vi "符合分析1.4.vi"(5 "大于信号周期":dbl, 6 "length":dbl=60.0 format="%#_13g", 7 "小于信号周期":dbl=120000.0, 8 "min bin":i32=30, 9 "通道B":i32=7, 10 "通道A":i32=6, 11 "file path (dialog if empty)":path=path "D:/tdc/2017/TDC_.fee01._20240514_102433.noAmp_-30mV_multiple_csv.csv") -> (0 "abnormal":bool=TRUE, 1 "Fitting RMS":dbl=2818.43112473961, 2 "Fitting center":dbl=-2250.0, 3 "mean":dbl=-3850.769384392631 format="%0.2f")   [LabVIEW 2017]
uses:
  <vilib>/Utility/file.llb/Read Delimited Spreadsheet (DBL).vi
  <vilib>/Analysis/NI_AALBase.lvlib
panel:
  out "Numeric 2":dbl=5.712308982040112e+16 format="%#_20f"
  out "Numeric":dbl=5.7122985833787944e+16 format="%#_20f"
  out "数值":i32=308738
  out "大小":i32=129310
  out "Histogram 2":dynamicdata(graph)=[{"t0"=timestamp(25 s since 1904-01-01), "dt"=50.0, "Y"=array[20000 elements], "attributes"=variant("NI_ChannelName"=variant(string " (直方图)"), "NI_ExpIsRelativeTime"=variant(bool TRUE), "NI_ExpStartTimeStamp"=variant(timestamp timestamp(3799126030.6251626 s since 1904-01-01)), "NI_ExpTimeStamp"=variant(timestamp timestamp(3799126030.6251626 s since 1904-01-01)), "NI_ExpXDimension"=variant(string "BIN"), "NI_OriginalChannelName"=variant(string ""))}] caption="直方图"
  out "数组":dbl[](array[numeric])
  out "Waveform Graph 5":dbl[](graph)
  in  "禁用的索引 (列)":i32=1
  in  "window":dbl=10000.0 format="%#_13g"
  in  "intervals":i32=200
  in  "min":dbl=-50000.0 format="%#_13g"
  in  "max":dbl=50000.0 format="%#_13g"
  out "XY Graph":cluster{"X":dbl, "Y":dbl}[](graph)
  out "list":dbl[][](array[numeric])
  out "counter":dbl[](array[numeric])=[139102.0, 129310.0, 0.0, 0.0, 0.0, 0.0, 20298.0, 20029.0, 0.0, 0.0, 0.0, 0.0, 0.0, 0.0, 0.0, 0.0, 0.0, 0.0, 0.0, 0.0, 0.0, 0.0, 0.0, 0.0, 0.0, 0.0, 0.0, 0.0, 0.0, 0.0, 0.0, 0.0, 0.0, 0.0, 0.0, 0.0, 0.0, 0.0, 0.0, 0.0, 0.0, 0.0, 0.0, 0.0, 0.0, 0.0, 0.0, 0.0, 0.0, 0.0, 0.0, 0.0, 0.0, 0.0, 0.0, 0.0, 0.0, 0.0, 0.0, 0.0, 0.0, 0.0, 0.0, 0.0]
  out "size(s) 2":i32[](array[numeric])=[308739, 128]
  out "Waveform Graph 4":dbl[](graph)
  out "B_start":i32
  out "A_start":i32
  out "start":i32
  out "mean 2":dbl=-3580.325380501851 format="%0.2f"
  out "standard deviation 2":dbl=2102.674360008159 format="%0.2f"
  out "Sum of 3 Gaussians 2":T1(graph)=[{"X Values"=[-13750.0, -13250.0, -12750.0, -12250.0, -11750.0, -11250.0, -10750.0, -10250.0, -9750.0, -9250.0, -8750.0, -8250.0, -7750.0, -7250.0, -6750.0, -6250.0, -5750.0, -5250.0, -4750.0, -4250.0, -3750.0, -3250.0, -2750.0, -2250.0, -1750.0, -1250.0, -750.0, -250.0, 250.0, 750.0, 1250.0, 1750.0, 2250.0, 2750.0, 3250.0, 3750.0, 4250.0, 4750.0, 5250.0, 5750.0, 6250.0, 6750.0, 7250.0, 7750.0, 8250.0, 8750.0, 9250.0, 9750.0, 10250.0, 10750.0, 11250.0, 11750.0, 12250.0, 12750.0, 13250.0, 13750.0, 14250.0, 14750.0, 15250.0, 15750.0], "Histogram: h(x)"=[0.00020516896563452846, 0.0005879803951743795, 0.00162597544504643, 0.004338754526689241, 0.011171619539264068, 0.027756656713886607, 0.06654541404560899, 0.1539462339582165, 0.34365286320062033, 0.7402370601310521, 1.538585524549578, 3.0858330069334388, 5.972046190316014, 11.152541711235395, 20.096689123234196, 34.94420244889411, 58.63078530864886, 94.92404789337367, 148.2950819797982, 223.55130384724364, 325.18284479713714, 456.43401817417424, 618.1990653887884, 807.9391318829133, 1018.8937603390267, 1239.87847954737, 1455.892475846031, 1649.6030130849056, 1803.555623444127, 1902.740668671416, 1937.0, 1902.740668671416, 1803.555623444127, 1649.6030130849056, 1455.892475846031, 1239.87847954737, 1018.8937603390267, 807.9391318829133, 618.1990653887884, 456.43401817417424, 325.18284479713714, 223.55130384724364, 148.2950819797982, 94.92404789337367, 58.63078530864886, 34.94420244889411, 20.096689123234196, 11.152541711235395, 5.972046190316014, 3.0858330069334388, 1.538585524549578, 0.7402370601310521, 0.34365286320062033, 0.1539462339582165, 0.06654541404560899, 0.027756656713886607, 0.011171619539264068, 0.004338754526689241, 0.00162597544504643, 0.0005879803951743795]}, {"X Values"=[-49750.0, -49250.0, -48750.0, -48250.0, -47750.0, -47250.0, -46750.0, -46250.0, -45750.0, -45250.0, -44750.0, -44250.0, -43750.0, -43250.0, -42750.0, -42250.0, -41750.0, -41250.0, -40750.0, -40250.0, -39750.0, -39250.0, -38750.0, -38250.0, -37750.0, -37250.0, -36750.0, -36250.0, -35750.0, -35250.0, -34750.0, -34250.0, -33750.0, -33250.0, -32750.0, -32250.0, -31750.0, -31250.0, -30750.0, -30250.0, -29750.0, -29250.0, -28750.0, -28250.0, -27750.0, -27250.0, -26750.0, -26250.0, -25750.0, -25250.0, -24750.0, -24250.0, -23750.0, -23250.0, -22750.0, -22250.0, -21750.0, -21250.0, -20750.0, -20250.0, -19750.0, -19250.0, -18750.0, -18250.0, -17750.0, -17250.0, -16750.0, -16250.0, -15750.0, -15250.0, -14750.0, -14250.0, -13750.0, -13250.0, -12750.0, -12250.0, -11750.0, -11250.0, -10750.0, -10250.0, -9750.0, -9250.0, -8750.0, -8250.0, -7750.0, -7250.0, -6750.0, -6250.0, -5750.0, -5250.0, -4750.0, -4250.0, -3750.0, -3250.0, -2750.0, -2250.0, -1750.0, -1250.0, -750.0, -250.0, 250.0, 750.0, 1250.0, 1750.0, 2250.0, 2750.0, 3250.0, 3750.0, 4250.0, 4750.0, 5250.0, 5750.0, 6250.0, 6750.0, 7250.0, 7750.0, 8250.0, 8750.0, 9250.0, 9750.0, 10250.0, 10750.0, 11250.0, 11750.0, 12250.0, 12750.0, 13250.0, 13750.0, 14250.0, 14750.0, 15250.0, 15750.0, 16250.0, 16750.0, 17250.0, 17750.0, 18250.0, 18750.0, 19250.0, 19750.0, 20250.0, 20750.0, 21250.0, 21750.0, 22250.0, 22750.0, 23250.0, 23750.0, 24250.0, 24750.0, 25250.0, 25750.0, 26250.0, 26750.0, 27250.0, 27750.0, 28250.0, 28750.0, 29250.0, 29750.0, 30250.0, 30750.0, 31250.0, 31750.0, 32250.0, 32750.0, 33250.0, 33750.0, 34250.0, 34750.0, 35250.0, 35750.0, 36250.0, 36750.0, 37250.0, 37750.0, 38250.0, 38750.0, 39250.0, 39750.0, 40250.0, 40750.0, 41250.0, 41750.0, 42250.0, 42750.0, 43250.0, 43750.0, 44250.0, 44750.0, 45250.0, 45750.0, 46250.0, 46750.0, 47250.0, 47750.0, 48250.0, 48750.0, 49250.0, 49750.0], "Histogram: h(x)"=[0.0, 0.0, 0.0, 0.0, 0.0, 0.0, 0.0, 0.0, 0.0, 0.0, 0.0, 0.0, 0.0, 0.0, 0.0, 0.0, 0.0, 0.0, 0.0, 0.0, 0.0, 0.0, 0.0, 0.0, 0.0, 0.0, 0.0, 0.0, 0.0, 0.0, 0.0, 0.0, 0.0, 0.0, 0.0, 0.0, 0.0, 0.0, 0.0, 0.0, 0.0, 0.0, 0.0, 0.0, 0.0, 0.0, 0.0, 0.0, 0.0, 0.0, 0.0, 0.0, 0.0, 0.0, 0.0, 0.0, 0.0, 0.0, 0.0, 0.0, 0.0, 0.0, 0.0, 0.0, 0.0, 0.0, 0.0, 0.0, 0.0, 0.0, 0.0, 0.0, 0.0, 0.0, 0.0, 0.0, 0.0, 0.0, 0.0, 0.0, 0.0, 0.0, 0.0, 0.0, 0.0, 0.0, 0.0, 134.0, 159.0, 231.0, 266.0, 307.0, 362.0, 464.0, 641.0, 831.0, 939.0, 1186.0, 1365.0, 1561.0, 1704.0, 1905.0, 1937.0, 1897.0, 1825.0, 1421.0, 313.0, 0.0, 0.0, 0.0, 0.0, 0.0, 0.0, 0.0, 0.0, 0.0, 0.0, 0.0, 0.0, 0.0, 0.0, 0.0, 0.0, 0.0, 0.0, 0.0, 0.0, 0.0, 0.0, 0.0, 0.0, 0.0, 0.0, 0.0, 0.0, 0.0, 0.0, 0.0, 0.0, 0.0, 0.0, 0.0, 0.0, 0.0, 0.0, 0.0, 0.0, 0.0, 0.0, 0.0, 0.0, 0.0, 0.0, 0.0, 0.0, 0.0, 0.0, 0.0, 0.0, 0.0, 0.0, 0.0, 0.0, 0.0, 0.0, 0.0, 0.0, 0.0, 0.0, 0.0, 0.0, 0.0, 0.0, 0.0, 0.0, 0.0, 0.0, 0.0, 0.0, 0.0, 0.0, 0.0, 0.0, 0.0, 0.0, 0.0, 0.0, 0.0, 0.0, 0.0, 0.0, 0.0, 0.0, 0.0, 0.0, 0.0, 0.0, 0.0, 0.0, 0.0]}]
  out "Fitting center 2":dbl=1250.0
  out "Fitting RMS 2":dbl=2646.6453634414506
  in  "min bin 2":i32=30
  in  "length 2":dbl=60.0 format="%#_13g"
  out "Waveform Graph 3":dbl[](graph)
  out "Waveform Graph 2":dbl[](graph)
  out "Sum of 3 Gaussians":T1(graph)=[{"X Values"=[-17250.0, -16750.0, -16250.0, -15750.0, -15250.0, -14750.0, -14250.0, -13750.0, -13250.0, -12750.0, -12250.0, -11750.0, -11250.0, -10750.0, -10250.0, -9750.0, -9250.0, -8750.0, -8250.0, -7750.0, -7250.0, -6750.0, -6250.0, -5750.0, -5250.0, -4750.0, -4250.0, -3750.0, -3250.0, -2750.0, -2250.0, -1750.0, -1250.0, -750.0, -250.0, 250.0, 750.0, 1250.0, 1750.0, 2250.0, 2750.0, 3250.0, 3750.0, 4250.0, 4750.0, 5250.0, 5750.0, 6250.0, 6750.0, 7250.0, 7750.0, 8250.0, 8750.0, 9250.0, 9750.0, 10250.0, 10750.0, 11250.0, 11750.0, 12250.0], "Histogram: h(x)"=[0.0013656626400436554, 0.003455839817507884, 0.008474140067424075, 0.020135829745501498, 0.0463634004710291, 0.10344580667038393, 0.2236569294966776, 0.46857993149481575, 0.9512986254154174, 1.8714658745731036, 3.5676218402583713, 6.590336255723455, 11.796907998790784, 20.46259315061705, 34.39418356941237, 56.01975417683496, 88.41567178978539, 135.22256256877975, 200.4014830434576, 287.7958710191195, 400.4977172476056, 540.0666872618658, 705.7105220811543, 893.5886714395316, 1096.4291526227148, 1303.6330216489944, 1501.9725298165247, 1676.8742089667392, 1814.140166258101, 1901.8359447148478, 1932.0, 1901.8359447148478, 1814.140166258101, 1676.8742089667392, 1501.9725298165247, 1303.6330216489944, 1096.4291526227148, 893.5886714395316, 705.7105220811543, 540.0666872618658, 400.4977172476056, 287.7958710191195, 200.4014830434576, 135.22256256877975, 88.41567178978539, 56.01975417683496, 34.39418356941237, 20.46259315061705, 11.796907998790784, 6.590336255723455, 3.5676218402583713, 1.8714658745731036, 0.9512986254154174, 0.46857993149481575, 0.2236569294966776, 0.10344580667038393, 0.0463634004710291, 0.020135829745501498, 0.008474140067424075, 0.003455839817507884]}, {"X Values"=[-49750.0, -49250.0, -48750.0, -48250.0, -47750.0, -47250.0, -46750.0, -46250.0, -45750.0, -45250.0, -44750.0, -44250.0, -43750.0, -43250.0, -42750.0, -42250.0, -41750.0, -41250.0, -40750.0, -40250.0, -39750.0, -39250.0, -38750.0, -38250.0, -37750.0, -37250.0, -36750.0, -36250.0, -35750.0, -35250.0, -34750.0, -34250.0, -33750.0, -33250.0, -32750.0, -32250.0, -31750.0, -31250.0, -30750.0, -30250.0, -29750.0, -29250.0, -28750.0, -28250.0, -27750.0, -27250.0, -26750.0, -26250.0, -25750.0, -25250.0, -24750.0, -24250.0, -23750.0, -23250.0, -22750.0, -22250.0, -21750.0, -21250.0, -20750.0, -20250.0, -19750.0, -19250.0, -18750.0, -18250.0, -17750.0, -17250.0, -16750.0, -16250.0, -15750.0, -15250.0, -14750.0, -14250.0, -13750.0, -13250.0, -12750.0, -12250.0, -11750.0, -11250.0, -10750.0, -10250.0, -9750.0, -9250.0, -8750.0, -8250.0, -7750.0, -7250.0, -6750.0, -6250.0, -5750.0, -5250.0, -4750.0, -4250.0, -3750.0, -3250.0, -2750.0, -2250.0, -1750.0, -1250.0, -750.0, -250.0, 250.0, 750.0, 1250.0, 1750.0, 2250.0, 2750.0, 3250.0, 3750.0, 4250.0, 4750.0, 5250.0, 5750.0, 6250.0, 6750.0, 7250.0, 7750.0, 8250.0, 8750.0, 9250.0, 9750.0, 10250.0, 10750.0, 11250.0, 11750.0, 12250.0, 12750.0, 13250.0, 13750.0, 14250.0, 14750.0, 15250.0, 15750.0, 16250.0, 16750.0, 17250.0, 17750.0, 18250.0, 18750.0, 19250.0, 19750.0, 20250.0, 20750.0, 21250.0, 21750.0, 22250.0, 22750.0, 23250.0, 23750.0, 24250.0, 24750.0, 25250.0, 25750.0, 26250.0, 26750.0, 27250.0, 27750.0, 28250.0, 28750.0, 29250.0, 29750.0, 30250.0, 30750.0, 31250.0, 31750.0, 32250.0, 32750.0, 33250.0, 33750.0, 34250.0, 34750.0, 35250.0, 35750.0, 36250.0, 36750.0, 37250.0, 37750.0, 38250.0, 38750.0, 39250.0, 39750.0, 40250.0, 40750.0, 41250.0, 41750.0, 42250.0, 42750.0, 43250.0, 43750.0, 44250.0, 44750.0, 45250.0, 45750.0, 46250.0, 46750.0, 47250.0, 47750.0, 48250.0, 48750.0, 49250.0, 49750.0], "Histogram: h(x)"=[0.0, 0.0, 0.0, 0.0, 0.0, 0.0, 0.0, 0.0, 0.0, 0.0, 0.0, 0.0, 0.0, 1.0, 0.0, 0.0, 0.0, 0.0, 0.0, 0.0, 0.0, 0.0, 0.0, 0.0, 0.0, 0.0, 0.0, 0.0, 0.0, 0.0, 1.0, 0.0, 0.0, 1.0, 1.0, 1.0, 1.0, 1.0, 0.0, 1.0, 1.0, 1.0, 1.0, 1.0, 0.0, 0.0, 1.0, 2.0, 1.0, 1.0, 0.0, 0.0, 0.0, 0.0, 1.0, 1.0, 1.0, 0.0, 1.0, 2.0, 1.0, 4.0, 1.0, 3.0, 4.0, 10.0, 8.0, 8.0, 14.0, 15.0, 10.0, 20.0, 26.0, 33.0, 35.0, 56.0, 56.0, 63.0, 87.0, 104.0, 154.0, 187.0, 218.0, 273.0, 318.0, 371.0, 500.0, 667.0, 847.0, 984.0, 1219.0, 1374.0, 1610.0, 1718.0, 1922.0, 1932.0, 1914.0, 1772.0, 1297.0, 171.0, 0.0, 0.0, 0.0, 0.0, 0.0, 0.0, 0.0, 0.0, 0.0, 0.0, 0.0, 0.0, 0.0, 0.0, 0.0, 0.0, 0.0, 0.0, 0.0, 0.0, 0.0, 0.0, 0.0, 0.0, 0.0, 0.0, 0.0, 0.0, 0.0, 0.0, 0.0, 0.0, 0.0, 0.0, 0.0, 0.0, 0.0, 0.0, 0.0, 0.0, 0.0, 0.0, 0.0, 0.0, 0.0, 0.0, 0.0, 0.0, 0.0, 0.0, 0.0, 0.0, 0.0, 0.0, 0.0, 0.0, 0.0, 0.0, 0.0, 0.0, 0.0, 0.0, 0.0, 0.0, 0.0, 0.0, 0.0, 0.0, 0.0, 0.0, 0.0, 0.0, 0.0, 0.0, 0.0, 0.0, 0.0, 0.0, 0.0, 0.0, 0.0, 0.0, 0.0, 0.0, 0.0, 0.0, 0.0, 0.0, 0.0, 0.0, 0.0, 0.0, 0.0, 0.0, 0.0, 0.0, 0.0, 0.0, 0.0, 0.0]}]
  out "index":i32=312652
  out "Waveform Graph":dbl[](graph)
  out "standard deviation":dbl=2676.6984531949533 format="%0.2f"
  in  "time offset":dbl
  out "size(s)":i32=20029
  out "Histogram":dynamicdata(graph)=[{"t0"=timestamp(-49500 s since 1904-01-01), "dt"=1000.0, "Y"=[0.0, 0.0, 0.0, 0.0, 0.0, 0.0, 1.0, 0.0, 0.0, 0.0, 0.0, 0.0, 0.0, 0.0, 0.0, 1.0, 1.0, 2.0, 2.0, 1.0, 2.0, 2.0, 0.0, 3.0, 2.0, 0.0, 0.0, 2.0, 1.0, 3.0, 5.0, 4.0, 15.0, 15.0, 29.0, 30.0, 59.0, 91.0, 120.0, 190.0, 346.0, 486.0, 695.0, 1161.0, 1847.0, 2577.0, 3348.0, 3834.0, 3699.0, 1455.0, 0.0, 0.0, 0.0, 0.0, 0.0, 0.0, 0.0, 0.0, 0.0, 0.0, 0.0, 0.0, 0.0, 0.0, 0.0, 0.0, 0.0, 0.0, 0.0, 0.0, 0.0, 0.0, 0.0, 0.0, 0.0, 0.0, 0.0, 0.0, 0.0, 0.0, 0.0, 0.0, 0.0, 0.0, 0.0, 0.0, 0.0, 0.0, 0.0, 0.0, 0.0, 0.0, 0.0, 0.0, 0.0, 0.0, 0.0, 0.0, 0.0, 0.0], "attributes"=variant("NI_ChannelName"=variant(string " (直方图)"), "NI_ExpIsRelativeTime"=variant(bool TRUE), "NI_ExpStartTimeStamp"=variant(timestamp timestamp(3799126031.478904 s since 1904-01-01)), "NI_ExpTimeStamp"=variant(timestamp timestamp(3799126031.478904 s since 1904-01-01)), "NI_ExpXDimension"=variant(string "BIN"), "NI_OriginalChannelName"=variant(string ""))}]
  # "2746167990257163.5"
  # "2746167990257033.5"
  # "2746167990255549.5"
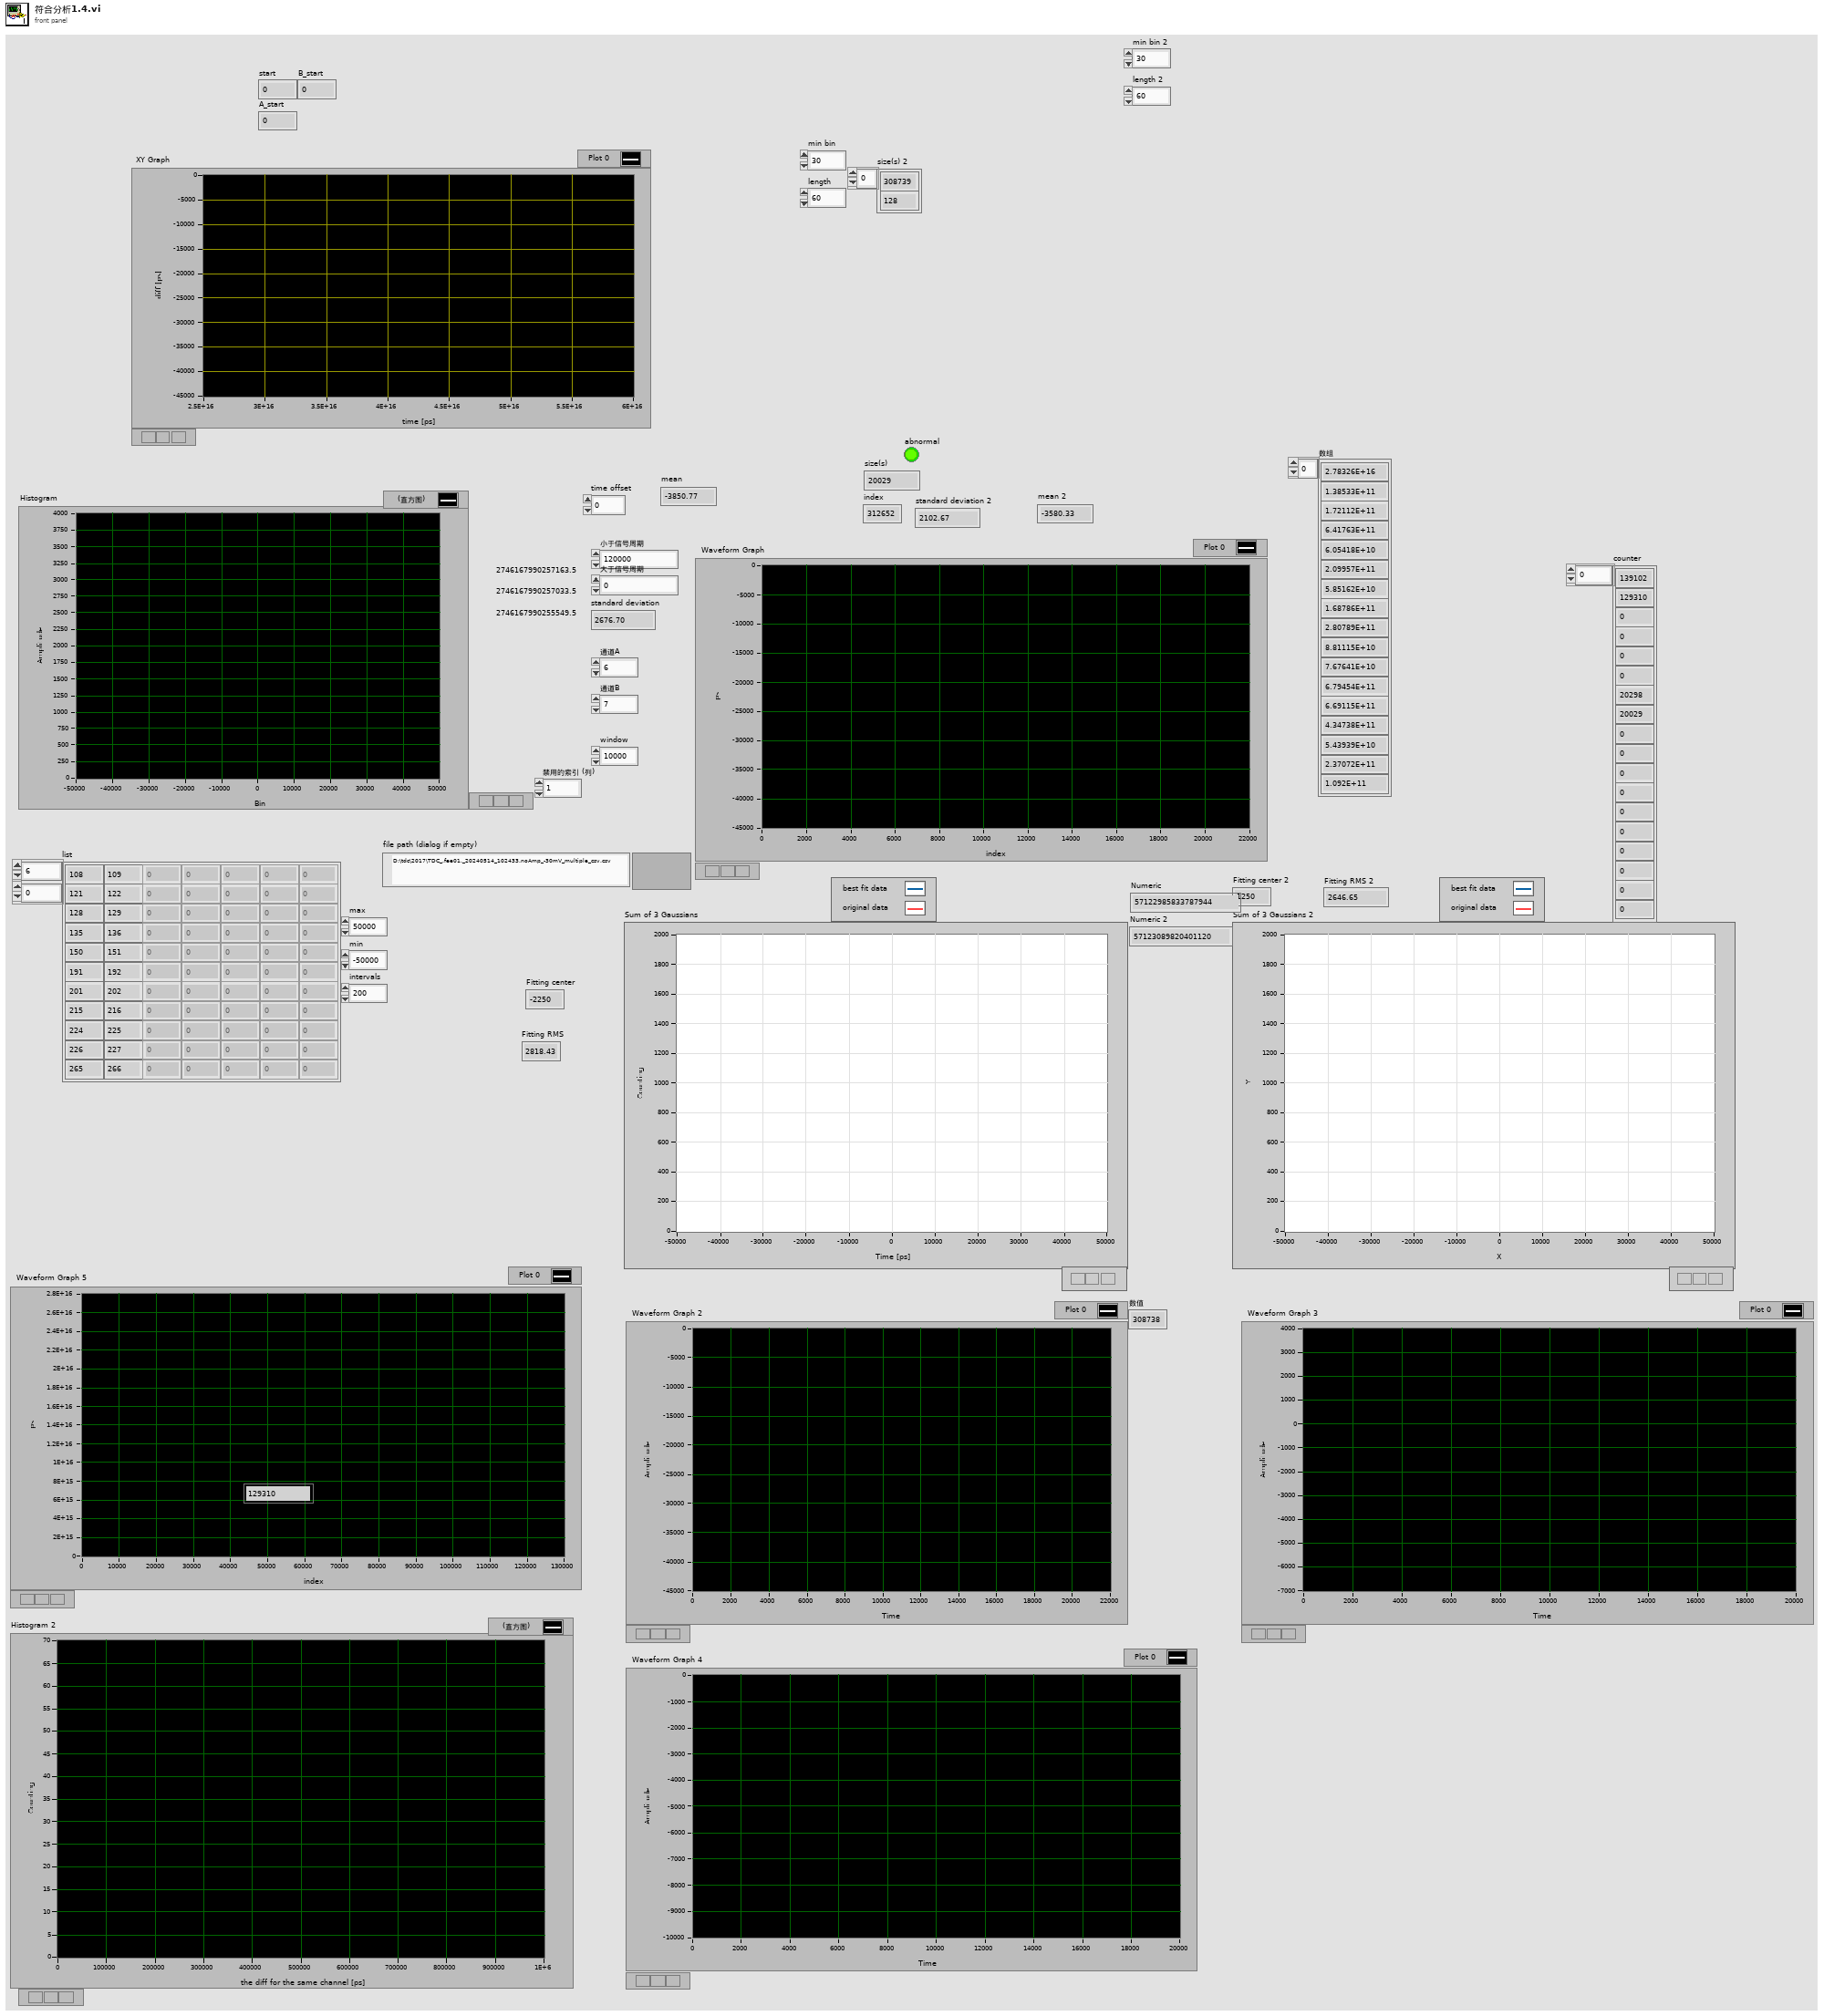
[diagram p1: front panel]
types:
  T1 = cluster{"X Values":dbl[], "Histogram: h(x)":dbl[]}[]
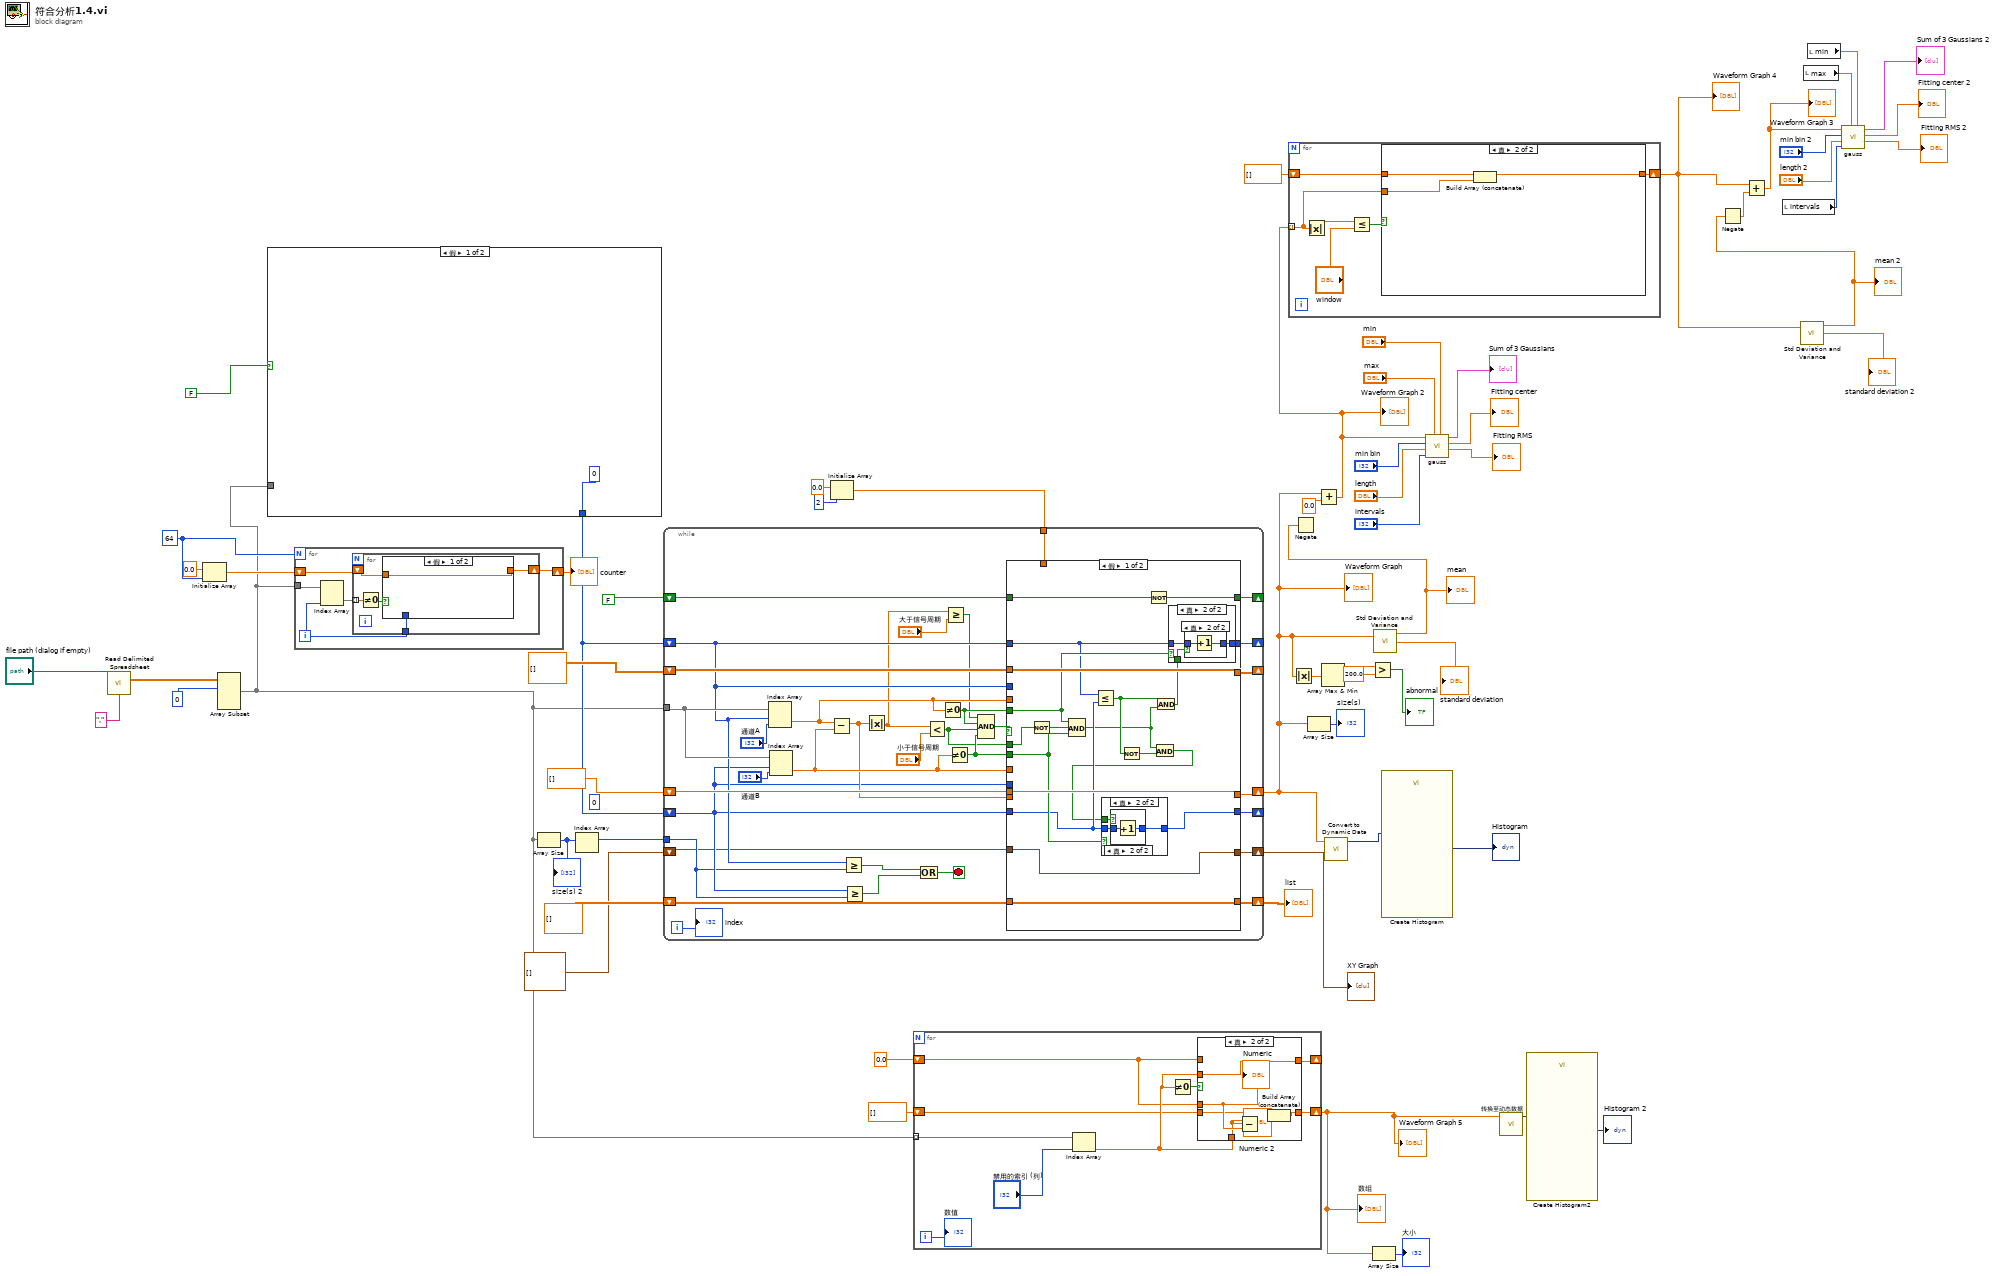
[diagram p0: block diagram]
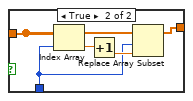
[diagram p3: hidden frame]
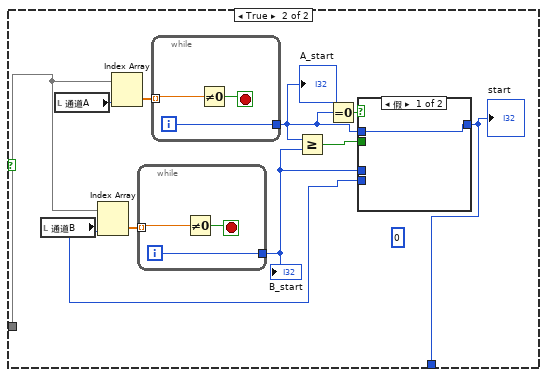
[diagram p4: hidden frame]
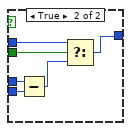
[diagram p5: hidden frame]
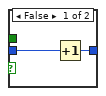
[diagram p7: hidden frame]
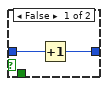
[diagram p9: hidden frame]
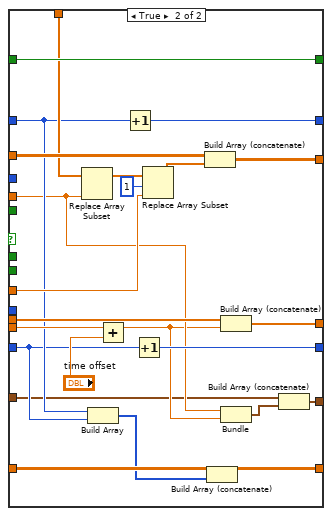
[diagram p11: hidden frame]
diagram:
  w23 = 64
  (unwired) 0
  n1 = call-poly <vilib>:"Read Delimited Spreadsheet.vi"("file path (dialog if empty)"="file path (dialog if empty)", "delimiter (\\t)"="," ("delimiter (\\t)")) -> ("all rows"=w57:dbl[][])  [unwired: 8 in, 5 out]
  n2 = Initialize Array(0.0 ("element"), w23) -> (w21:dbl[])
  n3 = Array Subset(array=w57, index (row)=0 ("length")) -> (w7:dbl[][])  [unwired: 3 in]
  n4 = case shown="假" FALSE {
    tunnel: w7 -> [_ w71]
    tunnel: [0 w69] -> w31
    frame False {
    }
    frame True {
      (unwired) 0
      n5 = local read "通道B"() -> (w67:i32)
      n6 = local read "通道A"() -> (w73:i32)
      n7 = Index Array(array=w71, index (col)=w67) -> (element=w72:dbl[])  [unwired: 1 in]
      n8 = Index Array(array=w71, index (col)=w73) -> (element=w74:dbl[])  [unwired: 1 in]
      n9 = while {
        tunnel: w72 -> [w84] mode=indexing
        tunnel: [w82] -> w68
        i -> [w82]
        stop <- w83 stop-if-true
        n10 = Not Equal To 0?(x=w84) -> (x != 0?=w83:bool)
      }
      "B_start" <- w68
      n11 = while {
        tunnel: w74 -> [w87] mode=indexing
        tunnel: [w85] -> w65
        i -> [w85]
        stop <- w86 stop-if-true
        n12 = Not Equal To 0?(x=w87) -> (x != 0?=w86:bool)
      }
      "A_start" <- w65
      n13 = Greater Or Equal?(x=w65, y=w68) -> (x >= y?=w70:bool)
      n14 = Equal To 0?(x=w65) -> (x = 0?=w66:bool)
      n15 = case shown="假" w66 {
        tunnel: w65 -> [w75 w81]
        tunnel: w70 -> [_ w80]
        tunnel: [w75 w79] -> w69
        tunnel: w68 -> [_ w78]
        tunnel: w67 -> [_ w76]
        frame False {
        }
        frame True {
          n16 = Subtract(x=w78, y=w76) -> (x-y=w77:i32)
          n17 = Select(t=w81, s=w80, f=w77) -> (s? t:f=w79:i32)
        }
      }
      "start" <- w69
    }
  }
  n18 = for {
    N: w23 -> [_]
    tunnel: w7 -> [w92]
    shift-right: [w88] -> w24
    shift-left: w21 -> [w90]
    i -> [w89]
    n19 = Index Array(array=w92, index (col)=w89) -> (element=w91:dbl[])  [unwired: 1 in]
    n20 = for {
      tunnel: w91 -> [w97] mode=indexing
      shift-right: [w93] -> w88
      shift-left: w90 -> [w96]
      tunnel: w89 -> [w95]
      n21 = Not Equal To 0?(x=w97) -> (x != 0?=w94:bool)
      n22 = case shown="假" w94 {
        tunnel: w96 -> [w98 w101]
        tunnel: w95 -> [_ w99]
        tunnel: [w98 w102] -> w93
        frame False {
        }
        frame True {
          n23 = Index Array(array=w101, index=w99) -> (element=w103:dbl)
          n24 = Increment(x=w103) -> (x+1=w100:dbl)
          n25 = Replace Array Subset(array=w101, new element=w100, index=w99) -> (w102:dbl[])
        }
      }
    }
  }
  "counter" <- w24
  n26 = Array Size(array=w7) -> (size(s)=w56:i32[])
  "size(s) 2" <- w56
  n27 = Index Array(array=w56) -> (element=w55:i32)  [unwired: 1 in]
  n28 = Initialize Array(0.0 ("element"), 2 ("dimension size")) -> (w58:dbl[])
  n29 = while {
    tunnel: w7 -> [w137]
    shift-right: [w133] -> _
    shift-left: w31 -> [w117]
    shift-right: [w130] -> _
    shift-left: w31 -> [w116]
    shift-right: [w131] -> _
    shift-left: FALSE -> [w132]
    shift-right: [w128] -> _
    shift-left: dbl[][] [] -> [w124]
    tunnel: w58 -> [w129]
    tunnel: w55 -> [w112]
    shift-right: [w120] -> w14
    shift-left: dbl[] [] -> [w119]
    shift-right: [w110] -> w8
    shift-left: dbl[][] [] -> [w109]
    shift-right: [w108] -> w18
    shift-left: cluster{"Numeric":dbl, dbl}[] [] -> [w107]
    i -> [w113]
    stop <- w125 stop-if-true
    n30 = Index Array(array=w137, index (row)=w117, index (col)="通道A") -> (element=w122:dbl)
    n31 = Index Array(array=w137, index (row)=w116, index (col)="通道B") -> (element=w121:dbl)
    n32 = Subtract(x=w122, y=w121) -> (x-y=w118:dbl)
    n33 = Greater Or Equal?(x=w117, y=w112) -> (x >= y?=w126:bool)
    n34 = Greater Or Equal?(x=w116, y=w112) -> (x >= y?=w127:bool)
    n35 = Absolute Value(x=w118) -> (abs(x)=w106:dbl)
    n36 = Compound Arithmetic op=OR(w126, w127) -> (w125:bool)
    n37 = Less?(x=w106, y="小于信号周期") -> (x < y?=w111:bool)
    n38 = Not Equal To 0?(x=w122) -> (x != 0?=w115:bool)
    n39 = Greater Or Equal?(x=w106, y="大于信号周期") -> (x >= y?=w104:bool)
    n40 = Not Equal To 0?(x=w121) -> (x != 0?=w114:bool)
    n41 = Compound Arithmetic op=AND(w104, w115, w111, w114) -> (w123:bool)
    n42 = case shown="假" w123 {
      tunnel: w117 -> [w143 w180]
      tunnel: [w156 w189] -> w133
      tunnel: w132 -> [w155 w196]
      tunnel: [w154 w196] -> w131
      tunnel: w116 -> [w144 w179]
      tunnel: [w151 w188] -> w130
      tunnel: w124 -> [w153 w195]
      tunnel: w129 -> [_ w194]
      tunnel: w122 -> [_ w177]
      tunnel: w121 -> [_ w183]
      tunnel: [w153 w190] -> w128
      tunnel: [w152 w187] -> w120
      tunnel: w119 -> [w152 w186]
      tunnel: w118 -> [_ w185]
      tunnel: w117 -> [_ _]
      tunnel: w116 -> [_ _]
      tunnel: w115 -> [w150 _]
      tunnel: w114 -> [w149 _]
      tunnel: w111 -> [w148 _]
      tunnel: [w146 w182] -> w110
      tunnel: w109 -> [w146 w181]
      tunnel: [w138 w174] -> w108
      tunnel: w107 -> [w138 w173]
      frame False {
        n43 = Not(x=w148) -> (.not. x?=w147:bool)
        n44 = Compound Arithmetic op=AND(w150, w147, w149) -> (w140:bool)
        n45 = Less Or Equal?(x=w143, y=w144) -> (x <= y?=w141:bool)
        n46 = Not(x=w141) -> (.not. x?=w142:bool)
        n47 = Not(x=w155) -> (.not. x?=w154:bool)
        n48 = And(x=w140, y=w142) -> (x .and. y?=w139:bool)
        n49 = case shown="真" w149 {
          tunnel: w144 -> [w158 w161]
          tunnel: [w157 w160] -> w151
          tunnel: w139 -> [_ w159]
          frame False {
            n50 = Increment(x=w158) -> (x+1=w157:i32)
          }
          frame True {
            n51 = case shown="真" w159 {
              tunnel: w161 -> [w162 w164]
              tunnel: [w162 w163] -> w160
              frame False {
              }
              frame True {
                n52 = Increment(x=w164) -> (x+1=w163:i32)
              }
            }
          }
        }
        n53 = And(x=w141, y=w140) -> (x .and. y?=w145:bool)
        n54 = case shown="真" w150 {
          tunnel: w143 -> [w166 w169]
          tunnel: [w165 w168] -> w156
          tunnel: w145 -> [_ w167]
          frame False {
            n55 = Increment(x=w166) -> (x+1=w165:i32)
          }
          frame True {
            n56 = case shown="真" w167 {
              tunnel: w169 -> [w170 w172]
              tunnel: [w170 w171] -> w168
              frame False {
              }
              frame True {
                n57 = Increment(x=w172) -> (x+1=w171:i32)
              }
            }
          }
        }
      }
      frame True {
        n58 = Replace Array Subset(array=w194, new element=w177) -> (w193:dbl[])  [unwired: 1 in]
        n59 = Build Array(w180, w179) -> (w178:i32[])
        n60 = Add(x=w185, y="time offset") -> (x+y=w176:dbl)
        n61 = Increment(x=w180) -> (x+1=w189:i32)
        n62 = Increment(x=w179) -> (x+1=w188:i32)
        n63 = Replace Array Subset(array=w193, new element=w183, index=1) -> (w191:dbl[])
        n64 = Build Array (concatenate)(w195, w191) -> (w190:dbl[][])
        n65 = Build Array (concatenate)(w181, w178) -> (w182:dbl[][])
        n66 = Build Array (concatenate)(w186, w176) -> (w187:dbl[])
        n67 = Bundle("Numeric"=w177, w176) -> (w175:cluster{"Numeric":dbl, dbl})  [unwired: 1 in]
        n68 = Build Array (concatenate)(w173, w175) -> (w174:cluster{"Numeric":dbl, dbl}[])
      }
    }
    "index" <- w113
  }
  "Waveform Graph" <- w14
  "list" <- w8
  "XY Graph" <- w18
  n69 = for {
    tunnel: w7 -> [w205] mode=indexing
    shift-right: [w203] -> _
    shift-left: 0.0 ("Numeric") -> [w198]
    shift-right: [w200] -> w2
    shift-left: dbl[] [] -> [w201]
    i -> [w197]
    n70 = Index Array(array=w205, index="禁用的索引 (列)") -> (element=w202:dbl)
    n71 = Not Equal To 0?(x=w202) -> (x != 0?=w204:bool)
    n72 = case shown="真" w204 {
      tunnel: w202 -> [_ w213]
      tunnel: [w207 w213] -> w203
      tunnel: w198 -> [w207 _]
      tunnel: w198 -> [_ w212]
      tunnel: w202 -> [_ w211]
      tunnel: w201 -> [w206 w209]
      tunnel: [w206 w208] -> w200
      frame False {
      }
      frame True {
        n73 = Subtract(x=w211, y=w212) -> (x-y=w210:dbl)
        n74 = Build Array (concatenate)(w209, w210) -> (w208:dbl[])
        "Numeric" <- w212
        "Numeric 2" <- w211
      }
    }
    "数值" <- w197
  }
  "Waveform Graph 5" <- w2
  "数组" <- w2
  n75 = Absolute Value(x=w14) -> (abs(x)=w29:dbl[])
  n76 = Array Size(array=w14) -> (size(s)=→"size(s)":i32)
  n77 = Add(x=w14, y=0.0) -> (x+y=w13:dbl[])
  "Waveform Graph 2" <- w13
  n78 = for {
    tunnel: w13 -> [w218] mode=indexing
    shift-right: [w216] -> w25
    shift-left: dbl[] [] -> [w217]
    n79 = Absolute Value(x=w218) -> (abs(x)=w214:dbl)
    n80 = Less Or Equal?(x=w214, y="window") -> (x <= y?=w219:bool)
    n81 = case shown="真" w219 {
      tunnel: w218 -> [_ w222]
      tunnel: w217 -> [w220 w223]
      tunnel: [w220 w221] -> w216
      frame False {
      }
      frame True {
        n82 = Build Array (concatenate)(w223, w222) -> (w221:dbl[])
      }
    }
  }
  "Waveform Graph 4" <- w25
  n83 = Array Max & Min(array=w29) -> (max value=w28:dbl)  [unwired: 3 out]
  n84 = call "Convert to Dynamic Data"("Array"=w14) -> ("Dynamic Data Type"=w51:dynamicdata)  [unwired: 3 in]
  n85 = Greater?(x=w28, y=200.0) -> (0:→"abnormal":bool)
  n86 = Array Size(array=w2) -> (size(s)=→"大小":i32)
  n87 = call <vilib>:"Std Deviation and Variance.vi"("X"=w14) -> ("mean"=w43:dbl, "standard deviation"=→"standard deviation":dbl)  [unwired: 1 in, 1 out]
  "mean" <- w43
  n88 = Negate(x=w43) -> ()  [unwired: 1 out]
  n89 = call "Create Histogram"("Signal"=w51) -> ("Histogram"=→"Histogram":dynamicdata)  [unwired: 9 in, 1 out]
  n90 = call "gauss.vi"("min"="min", "max"="max", "intervals"="intervals", "length"="length", "low"="min bin", "Waveform Graph"=w13) -> ("standard deviation"=→"Fitting RMS":dbl, "center"=→"Fitting center":dbl, "Sum of 3 Gaussians"=→"Sum of 3 Gaussians":T1)  [unwired: 3 in]
  n91 = call "转换至动态数据"("Array"=w2) -> ("Dynamic Data Type"=w4:dynamicdata)  [unwired: 3 in]
  n92 = call "Create Histogram2"("Signal"=w4) -> ("Histogram"=→"Histogram 2":dynamicdata)  [unwired: 9 in, 1 out]
  n93 = local read "intervals"() -> (w10:i32)
  n94 = call <vilib>:"Std Deviation and Variance.vi"("X"=w25) -> ("mean"=w33:dbl, "standard deviation"=→"standard deviation 2":dbl)  [unwired: 1 in, 1 out]
  "mean 2" <- w33
  n95 = Negate(x=w33) -> (-x=w40:dbl)
  n96 = Add(x=w25, y=w40) -> (x+y=w41:dbl[])
  "Waveform Graph 3" <- w41
  n97 = local read "max"() -> (w11:dbl)
  n98 = local read "min"() -> (w12:dbl)
  n99 = call "gauss.vi"("min"=w12, "max"=w11, "intervals"=w10, "length"="length 2", "low"="min bin 2", "Waveform Graph"=w41) -> ("standard deviation"=→"Fitting RMS 2":dbl, "center"=→"Fitting center 2":dbl, "Sum of 3 Gaussians"=→"Sum of 3 Gaussians 2":T1)  [unwired: 3 in]
